vi "Lift.vi"(0 "LiftLocation":T1(ring)) -> ()   [LabVIEW 2018]
uses:
  <vilib>/Rock Robotics/SystemInterfaces/DIO/FPGA_DIOChannel.ctl
  <vilib>/Rock Robotics/WPI/ThirdParty/Phoenix-LabVIEW/Motor Controller/Controls/CTRE_Phoenix_MotorControl_ControlMode.ctl
  Lift Global.vi
  Times/Times Global.vi
  <vilib>/addons/control/pid/pid.llb/PID (DBL).vi
  <vilib>/Rock Robotics/WPI/ThirdParty/Phoenix-LabVIEW/Motor Controller/Get/CTRE_Phoenix_MotorController_GetSelectedSensorData.vi
  Cargo Intake/Cargo Intake Global.vi
  <vilib>/addons/control/pid/NI_PID_pid.lvlib
panel:
  in  "Output Scalar":dbl=0.6 format="%#_13g"
  in  "t":dbl=0.6 format="%#_13g"
  in  "output range":cluster{"output high":dbl, "output low":dbl}={"output high"=1.0, "output low"=-1.0}
  in  "LiftMode":T2(ring)=enum."Basic Control"
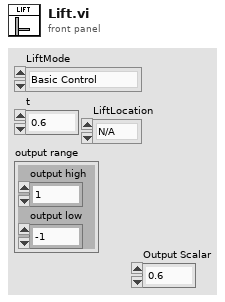
[diagram p1: front panel]
types:
  T1 = enum16{"N/A", "Hatch Panel Zone 1", "Hatch Panel Zone 2", "Hatch Panel Zone 3", "Cargo Zone 1", "Cargo Zone 2", "Cargo Zone 3"}
  T2 = enum16{"Ultra Manual Control", "Manual Control", "Basic Control", "Automated Control", "Autonomous Control"}
  T3 = typedef "FPGA_DIOChannel.ctl" = enum8{"DIO 0", "DIO 1", "DIO 2", "DIO 3", "DIO 4", "DIO 5", "DIO 6", "DIO 7", "DIO 8", "DIO 9", "DIO MXP 0", "DIO MXP 1", "DIO MXP 2", "DIO MXP 3", "DIO MXP 4", "DIO MXP 5", "DIO MXP 6", "DIO MXP 7", "DIO MXP 8", "DIO MXP 9", "DIO MXP 10", "DIO MXP 11", "DIO MXP 12", "DIO MXP 13", "DIO MXP 14", "DIO MXP 15", "SPI Port CS1", "SPI Port CS2", "SPI Port CS3", "SPI Port MISO", "SPI Port MOSI", "Invalid"}
  T4 = typedef "WPI_DigitalInputDevRef.ctl" = cluster{"DevStatus":errorcluster, "DIO Channel":T3}
  T5 = typedef "WPI_MotorControlDeviceRef.ctl" = cluster{"DeviceStatus":errorcluster, "Type":T6, "PWM":cluster{"PWM Channel":T7, "DeadBand":T8}, "CAN":cluster{"Device Number":u8, "SetOutput VI Ref":variant, "GetOutput VI Ref":variant, "Enable VI Ref":variant, "Disable VI Ref":variant, "Data":variant}, "Invert":bool, "DIO PWM":cluster{"PWM \"Enable\" Channel":T7, "DIOChannel":T3, "PWM Rate":dbl}}
  T6 = typedef "WPI_MotorControlType.ctl" = enum16{"PWM", "CAN", "DIO PWM"}
  T7 = typedef "FPGA_DIOPWMChannel.ctl" = enum8{"PWM 0", "PWM 1", "PWM 2", "PWM 3", "PWM 4", "PWM 5", "PWM 6", "PWM 7", "PWM 8", "PWM 9", "PWM MXP 0", "PWM MXP 1", "PWM MXP 2", "PWM MXP 3", "PWM MXP 4", "PWM MXP 5", "PWM MXP 6", "PWM MXP 7", "PWM MXP 8", "PWM MXP 9", "Invalid"}
  T8 = typedef "WPI_PWMDeadband.ctl" = cluster{"Name":string, "maxPositivePwm":i32, "minPositivePwm":i32, "centerPwm":i32, "maxNegativePwm":i32, "minNegativePwm":i32, "angularRange":u16}
  T9 = typedef "CTRE_Phoenix_MotorControl_ControlMode.ctl" = u16
  T10 = typedef "Control 3.ctl" = dbl
  T11 = cluster{"proportional gain (Kc)":dbl, "integral time(Ti, min)":dbl, "derivative time(Td, min) 2":dbl}
  T12 = enum16{"Hatch Panel Zone 1", "Hatch Panel Zone 2", "Hatch Panel Zone 3", "Cargo Zone 1", "Cargo Zone 2", "Cargo Zone 3", "Cargo Ship Zone"}
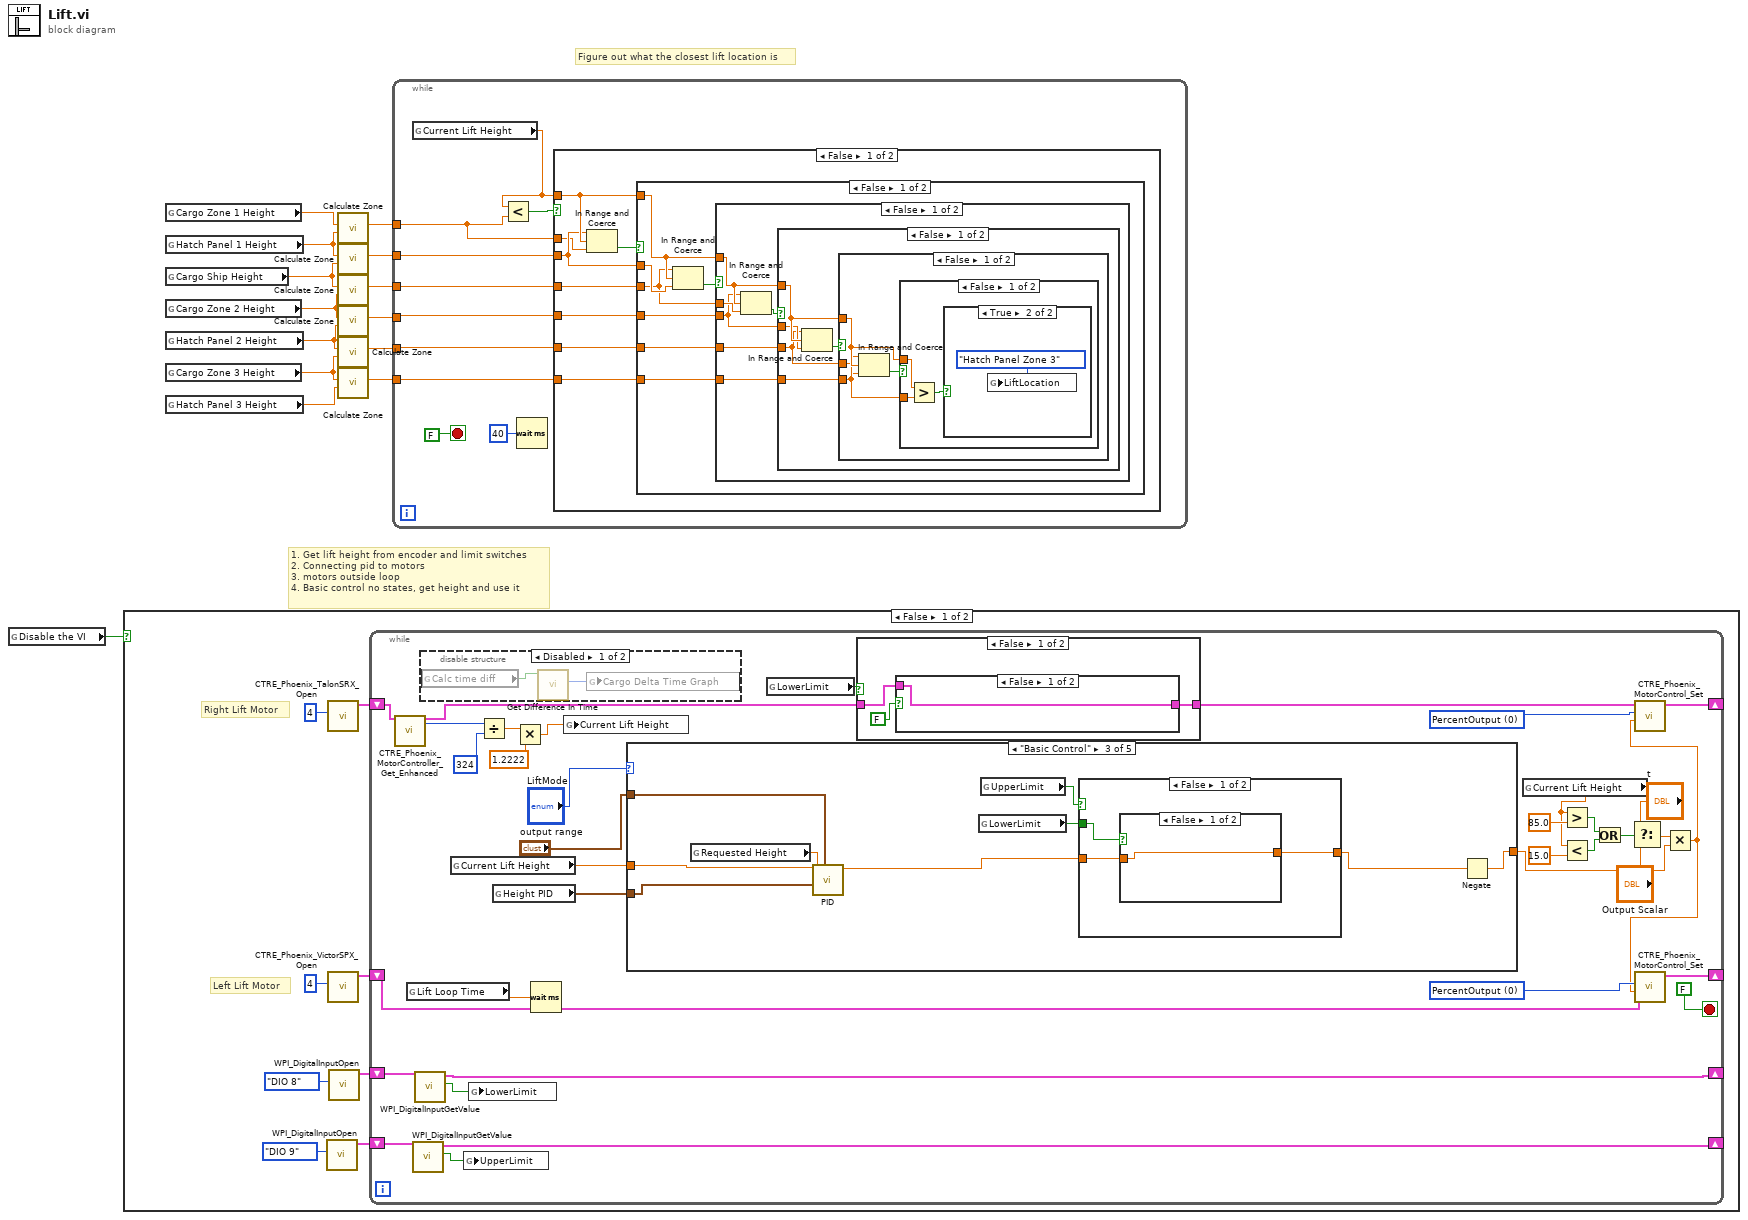
[diagram p0: block diagram]
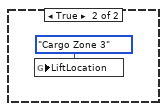
[diagram p3: hidden frame]
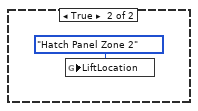
[diagram p4: hidden frame]
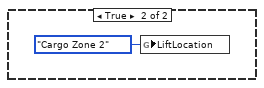
[diagram p5: hidden frame]
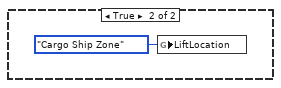
[diagram p6: hidden frame]
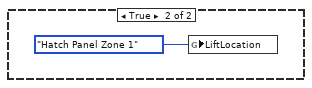
[diagram p7: hidden frame]
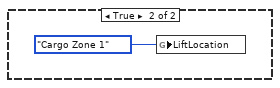
[diagram p8: hidden frame]
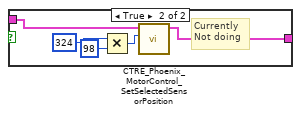
[diagram p9: hidden frame]
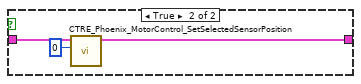
[diagram p10: hidden frame]
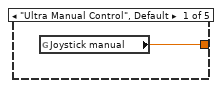
[diagram p12: hidden frame]
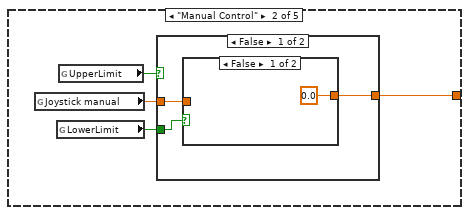
[diagram p13: hidden frame]
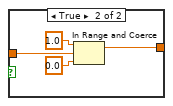
[diagram p14: hidden frame]
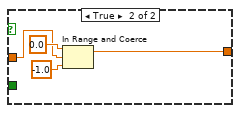
[diagram p15: hidden frame]
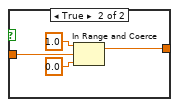
[diagram p16: hidden frame]
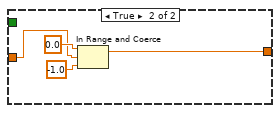
[diagram p17: hidden frame]
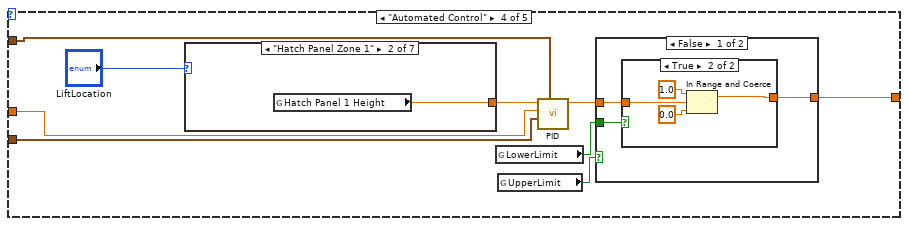
[diagram p18: hidden frame]
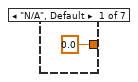
[diagram p19: hidden frame]
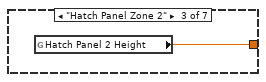
[diagram p20: hidden frame]
diagram:
  # "Figure out what the closest lift location is"
  # "1. Get lift height from encoder and limit switches\n2. Connecting pid to motors\n3. motors outside loop\n4. Basic control no states, get height and use it"
  n1 = global read "Lift Global.vi" "Disable the VI"() -> (w14:bool)
  n2 = case shown="False" w14 {
    frame False {
      # "Left Lift Motor"
      # "Right Lift Motor"
      n3 = call <vilib>:"WPI_DigitalInputOpen.vi"("DIO Channel"=FPGA_DIOChannel."DIO 9") -> ("DigitalInputDevRef"=w15:T4)  [unwired: 9 in, 1 out]
      n4 = call <vilib>:"CTRE_Phoenix_TalonSRX_Open.vi"("Device Number"=u8 4) -> ("CAN Talon SRX Ref"=w22:T5)  [unwired: 9 in, 1 out]
      n5 = call <vilib>:"CTRE_Phoenix_VictorSPX_Open.vi"("Device Number"=u8 4) -> ("CAN Talon SRX Ref"=w20:T5)  [unwired: 9 in, 1 out]
      n6 = call <vilib>:"WPI_DigitalInputOpen.vi"("DIO Channel"=FPGA_DIOChannel."DIO 8") -> ("DigitalInputDevRef"=w17:T4)  [unwired: 9 in, 1 out]
      n7 = while {
        shift-right: [w55] -> _
        shift-left: w22 -> [w48]
        shift-right: [w53] -> _
        shift-left: w20 -> [w52]
        shift-right: [w42] -> _
        shift-left: w17 -> [w43]
        shift-right: [w37] -> _
        shift-left: w15 -> [w38]
        stop <- FALSE stop-if-true
        w54 = T9 0 items=["PercentOutput"=0, "Position"=1, "Velocity"=2, "Current"=3, "Follower"=5, "MotionProfile"=6, "MotionMagic"=7, "MotionProfileArc"=10, "Disabled"=15] ("Control Mode")
        w56 = T9 0 items=["PercentOutput"=0, "Position"=1, "Velocity"=2, "Current"=3, "Follower"=5, "MotionProfile"=6, "MotionMagic"=7, "MotionProfileArc"=10, "Disabled"=15] ("Control Mode")
        n8 = call-poly <vilib>:"CTRE_Phoenix_MotorController_Get_Enhanced.vi"("PhoenixMotorControlDevRef"=w48) -> ("PhoenixMotorControlDevRef"=w47:T5, "Position (Raw Sensor Units)"=w45:i32)  [unwired: 11 in, 2 out]
        n9 = global read "Times Global.vi" "Lift Loop Time"() -> (w59:T10)
        n10 = call <vilib>:"WPI_DigitalInputGetValue.vi"("DigitalInputDevRef"=w38) -> ("Value"=w40:bool, "DigitalInputDevRef"=w37:T4)  [unwired: 8 in, 1 out]
        n11 = call <vilib>:"WPI_DigitalInputGetValue.vi"("DigitalInputDevRef"=w43) -> ("Value"=w41:bool, "DigitalInputDevRef"=w42:T4)  [unwired: 8 in, 1 out]
        n12 = disable-structure shown="Disabled" {
          frame Disabled {
            n13 = global read "Cargo Intake Global.vi" "Calc time diff"() -> (w73:bool)
            n14 = call "Get Difference In Time.vi"("Calculate Time Difference"=w73) -> ("Delta Time over Time"=w72:u32)  [unwired: 9 in, 1 out]
            n15 = global write "Times Global.vi" "Cargo Delta Time Graph"(w72) -> ()
          }
          frame Enabled {
          }
        }
        n16 = global read "Lift Global.vi" "Current Lift Height"() -> (w49:dbl)
        n17 = global write "Lift Global.vi" "UpperLimit"(w40) -> ()
        n18 = global write "Lift Global.vi" "LowerLimit"(w41) -> ()
        n19 = Divide(x=w45, y=324) -> (x/y=w25:dbl)
        n20 = global read "Lift Global.vi" "Height PID"() -> (w50:T11)
        n21 = Multiply(x=w25, y=1.2222) -> (x*y=w24:dbl)
        n22 = Wait (ms)(milliseconds to wait=w59) -> ()  [unwired: 1 out]
        n23 = global write "Lift Global.vi" "Current Lift Height"(w24) -> ()
        n24 = case shown="\"Basic Control\"" "LiftMode" {
          tunnel: [w74 w75 w95 w117 0.0 ("Cargo Zone 3 Height")] -> w29
          tunnel: w49 -> [_ _ w99 w115 _]
          tunnel: w50 -> [_ _ w98 w114 _]
          tunnel: "output range" -> [_ _ w97 w116 _]
          frame "Ultra Manual Control", Default {
            n25 = global read "Lift Global.vi" "Joystick manual"() -> (w74:dbl)
          }
          frame "Manual Control" {
            n26 = global read "Lift Global.vi" "Joystick manual"() -> (w76:dbl)
            n27 = global read "Lift Global.vi" "LowerLimit"() -> (w78:bool)
            n28 = global read "Lift Global.vi" "UpperLimit"() -> (w77:bool)
            n29 = case shown="False" w77 {
              tunnel: w78 -> [w81 _]
              tunnel: [w80 w88] -> w75
              tunnel: w76 -> [w79 w87]
              frame False {
                n30 = case shown="False" w81 {
                  tunnel: [0.0 w86] -> w80
                  tunnel: w79 -> [_ w83]
                  frame False {
                  }
                  frame True {
                    n31 = In Range and Coerce(upper limit=1.0, x=w83, lower limit=0.0) -> (coerced(x)=w86:dbl)  [unwired: 1 out]
                  }
                }
              }
              frame True {
                n32 = In Range and Coerce(upper limit=0.0, x=w87, lower limit=-1.0) -> (coerced(x)=w88:dbl)  [unwired: 1 out]
              }
            }
          }
          frame "Basic Control" {
            n33 = global read "Lift Global.vi" "Requested Height"() -> (w96:dbl)
            n34 = call-poly <vilib>:"PID.vi"("output range"=w97, "PID gains"=w98, "process variable"=w99, "setpoint"=w96) -> ("output"=w92:dbl)  [unwired: 6 in, 1 out]
            n35 = global read "Lift Global.vi" "LowerLimit"() -> (w94:bool)
            n36 = global read "Lift Global.vi" "UpperLimit"() -> (w93:bool)
            n37 = case shown="False" w93 {
              tunnel: w94 -> [w102 _]
              tunnel: [w101 w109] -> w91
              tunnel: w92 -> [w100 w108]
              frame False {
                n38 = case shown="False" w102 {
                  tunnel: [w103 w107] -> w101
                  tunnel: w100 -> [w103 w104]
                  frame False {
                  }
                  frame True {
                    n39 = In Range and Coerce(upper limit=1.0, x=w104, lower limit=0.0) -> (coerced(x)=w107:dbl)  [unwired: 1 out]
                  }
                }
              }
              frame True {
                n40 = In Range and Coerce(upper limit=0.0, x=w108, lower limit=-1.0) -> (coerced(x)=w109:dbl)  [unwired: 1 out]
              }
            }
            n41 = Negate(x=w91) -> (-x=w95:dbl)
          }
          frame "Automated Control" {
            n42 = case shown="\"Hatch Panel Zone 1\"" "LiftLocation" {
              tunnel: [0.0 ("Cargo Zone 3 Height") w122 w123 w124 w125 w126 w127] -> w112
              frame "N/A", Default {
              }
              frame "Hatch Panel Zone 1" {
                n43 = global read "Lift Global.vi" "Hatch Panel 1 Height"() -> (w122:dbl)
              }
              frame "Hatch Panel Zone 2" {
                n44 = global read "Lift Global.vi" "Hatch Panel 2 Height"() -> (w123:dbl)
              }
              frame "Hatch Panel Zone 3" {
                n45 = global read "Lift Global.vi" "Hatch Panel 3 Height"() -> (w124:dbl)
              }
              frame "Cargo Zone 1" {
                n46 = global read "Lift Global.vi" "Cargo Zone 1 Height"() -> (w125:dbl)
              }
              frame "Cargo Zone 2" {
                n47 = global read "Lift Global.vi" "Cargo Zone 2 Height"() -> (w126:dbl)
              }
              frame "Cargo Zone 3" {
                n48 = global read "Lift Global.vi" "Cargo Zone 3 Height"() -> (w127:dbl)
              }
            }
            n49 = global read "Lift Global.vi" "LowerLimit"() -> (w120:bool)
            n50 = global read "Lift Global.vi" "UpperLimit"() -> (w119:bool)
            n51 = call-poly <vilib>:"PID.vi"("output range"=w116, "PID gains"=w114, "process variable"=w115, "setpoint"=w112) -> ("output"=w118:dbl)  [unwired: 6 in, 1 out]
            n52 = case shown="False" w119 {
              tunnel: w120 -> [w130 _]
              tunnel: [w129 w137] -> w117
              tunnel: w118 -> [w128 w136]
              frame False {
                n53 = case shown="True" w130 {
                  tunnel: [0.0 w135] -> w129
                  tunnel: w128 -> [_ w132]
                  frame False {
                  }
                  frame True {
                    n54 = In Range and Coerce(upper limit=1.0, x=w132, lower limit=0.0) -> (coerced(x)=w135:dbl)  [unwired: 1 out]
                  }
                }
              }
              frame True {
                n55 = In Range and Coerce(upper limit=0.0, x=w136, lower limit=-1.0) -> (coerced(x)=w137:dbl)  [unwired: 1 out]
              }
            }
          }
          frame "Autonomous Control" {
          }
        }
        n56 = global read "Lift Global.vi" "LowerLimit"() -> (w39:bool)
        n57 = case shown="False" w39 {
          tunnel: w47 -> [w62 w71]
          tunnel: [w61 w70] -> w46
          frame False {
            n58 = case shown="False" FALSE {
              tunnel: w62 -> [w63 w68]
              tunnel: [w63 w67] -> w61
              frame False {
              }
              frame True {
                # "Currently\nNot doing"
                n59 = Multiply(x=324 ("y"), y=98 ("New Sensor Position")) -> (x*y=w64:i32)
                n60 = call <vilib>:"CTRE_Phoenix_MotorControl_SetSelectedSensorPosition.vi"("New Sensor Position"=w64, "PhoenixMotorControlDevRef"=w68) -> ("PhoenixMotorControlDevRef"=w67:T5)  [unwired: 8 in, 1 out]
              }
            }
          }
          frame True {
            n61 = call <vilib>:"CTRE_Phoenix_MotorControl_SetSelectedSensorPosition.vi"("New Sensor Position"=0, "PhoenixMotorControlDevRef"=w71) -> ("PhoenixMotorControlDevRef"=w70:T5)  [unwired: 8 in, 1 out]
          }
        }
        n62 = global read "Lift Global.vi" "Current Lift Height"() -> (w34:dbl)
        n63 = Greater?(x=w34, y=85.0) -> (0:w32:bool)
        n64 = Less?(x=w34, y=15.0) -> (x < y?=w33:bool)
        n65 = Or(x=w32, y=w33) -> (x .or. y?=w31:bool)
        n66 = Select(t="t", s=w31, f="Output Scalar") -> (s? t:f=w30:dbl)
        n67 = Multiply(x=w30, y=w29) -> (x*y=w26:dbl)
        n68 = call <vilib>:"CTRE_Phoenix_MotorControl_Set.vi"("Output"=w26, "Control Mode"=w56, "PhoenixMotorControlDevRef"=w46) -> ("PhoenixMotorControlDevRef"=w55:T5)  [unwired: 7 in, 1 out]
        n69 = call <vilib>:"CTRE_Phoenix_MotorControl_Set.vi"("Output"=w26, "Control Mode"=w54, "PhoenixMotorControlDevRef"=w52) -> ("PhoenixMotorControlDevRef"=w53:T5)  [unwired: 7 in, 1 out]
      }
    }
    frame True {
    }
  }
  n70 = global read "Lift Global.vi" "Cargo Zone 1 Height"() -> (w7:dbl)
  n71 = global read "Lift Global.vi" "Hatch Panel 1 Height"() -> (w13:dbl)
  n72 = global read "Lift Global.vi" "Cargo Ship Height"() -> (w12:dbl)
  n73 = global read "Lift Global.vi" "Cargo Zone 2 Height"() -> (w11:dbl)
  n74 = global read "Lift Global.vi" "Hatch Panel 2 Height"() -> (w10:dbl)
  n75 = global read "Lift Global.vi" "Cargo Zone 3 Height"() -> (w9:dbl)
  n76 = global read "Lift Global.vi" "Hatch Panel 3 Height"() -> (w8:dbl)
  n77 = call "Calculate Zone.vi"("Top Height"=w13, "Bottom Height"=w7) -> ("Midpoint"=w6:dbl)  [unwired: 9 in]
  n78 = call "Calculate Zone.vi"("Top Height"=w12, "Bottom Height"=w13) -> ("Midpoint"=w5:dbl)  [unwired: 9 in]
  n79 = call "Calculate Zone.vi"("Top Height"=w11, "Bottom Height"=w12) -> ("Midpoint"=w4:dbl)  [unwired: 9 in]
  n80 = call "Calculate Zone.vi"("Top Height"=w10, "Bottom Height"=w11) -> ("Midpoint"=w3:dbl)  [unwired: 9 in]
  n81 = call "Calculate Zone.vi"("Top Height"=w9, "Bottom Height"=w10) -> ("Midpoint"=w2:dbl)  [unwired: 9 in]
  n82 = call "Calculate Zone.vi"("Top Height"=w8, "Bottom Height"=w9) -> ("Midpoint"=w1:dbl)  [unwired: 9 in]
  n83 = while {
    tunnel: w6 -> [w146]
    tunnel: w5 -> [w145]
    tunnel: w4 -> [w144]
    tunnel: w3 -> [w143]
    tunnel: w2 -> [w142]
    tunnel: w1 -> [w141]
    stop <- FALSE stop-if-true
    n84 = global read "Lift Global.vi" "Current Lift Height"() -> (w147:dbl)
    n85 = Less?(x=w147, y=w146) -> (x < y?=w148:bool)
    n86 = Wait (ms)(milliseconds to wait=u32 40) -> ()  [unwired: 1 out]
    n87 = case shown="False" w148 {
      tunnel: w147 -> [w154 _]
      tunnel: w146 -> [w152 _]
      tunnel: w145 -> [w153 _]
      tunnel: w144 -> [w158 _]
      tunnel: w143 -> [w157 _]
      tunnel: w142 -> [w156 _]
      tunnel: w141 -> [w155 _]
      frame False {
        n88 = In Range and Coerce(upper limit=w153, x=w154, lower limit=w152) -> (In Range?=w151:bool)  [unwired: 1 out]
        n89 = case shown="False" w151 {
          tunnel: w154 -> [w161 _]
          tunnel: w153 -> [w160 _]
          tunnel: w158 -> [w159 _]
          tunnel: w157 -> [w165 _]
          tunnel: w156 -> [w164 _]
          tunnel: w155 -> [w163 _]
          frame False {
            n90 = In Range and Coerce(upper limit=w159, x=w161, lower limit=w160) -> (In Range?=w162:bool)  [unwired: 1 out]
            n91 = case shown="False" w162 {
              tunnel: w161 -> [w168 _]
              tunnel: w165 -> [w166 _]
              tunnel: w164 -> [w171 _]
              tunnel: w163 -> [w170 _]
              tunnel: w159 -> [w167 _]
              frame False {
                n92 = In Range and Coerce(upper limit=w166, x=w168, lower limit=w167) -> (In Range?=w169:bool)  [unwired: 1 out]
                n93 = case shown="False" w169 {
                  tunnel: w168 -> [w174 _]
                  tunnel: w171 -> [w172 _]
                  tunnel: w170 -> [w176 _]
                  tunnel: w166 -> [w173 _]
                  frame False {
                    n94 = In Range and Coerce(upper limit=w172, x=w174, lower limit=w173) -> (In Range?=w175:bool)  [unwired: 1 out]
                    n95 = case shown="False" w175 {
                      tunnel: w174 -> [w179 _]
                      tunnel: w176 -> [w178 _]
                      tunnel: w172 -> [w177 _]
                      frame False {
                        n96 = In Range and Coerce(upper limit=w178, x=w179, lower limit=w177) -> (In Range?=w180:bool)  [unwired: 1 out]
                        n97 = case shown="False" w180 {
                          tunnel: w179 -> [w183 _]
                          tunnel: w178 -> [w182 _]
                          frame False {
                            n98 = Greater?(x=w183, y=w182) -> (0:w181:bool)
                            n99 = case shown="True" w181 {
                              frame False {
                              }
                              frame True {
                                n100 = global write "Lift Global.vi" "LiftLocation"(T12."Hatch Panel Zone 3" ("LiftLocation")) -> ()
                              }
                            }
                          }
                          frame True {
                            n101 = global write "Lift Global.vi" "LiftLocation"(T12."Cargo Zone 3" ("LiftLocation")) -> ()
                          }
                        }
                      }
                      frame True {
                        n102 = global write "Lift Global.vi" "LiftLocation"(T12."Hatch Panel Zone 2" ("LiftLocation")) -> ()
                      }
                    }
                  }
                  frame True {
                    n103 = global write "Lift Global.vi" "LiftLocation"(T12."Cargo Zone 2" ("LiftLocation")) -> ()
                  }
                }
              }
              frame True {
                n104 = global write "Lift Global.vi" "LiftLocation"(T12."Cargo Ship Zone" ("LiftLocation")) -> ()
              }
            }
          }
          frame True {
            n105 = global write "Lift Global.vi" "LiftLocation"(T12."Hatch Panel Zone 1" ("LiftLocation")) -> ()
          }
        }
      }
      frame True {
        n106 = global write "Lift Global.vi" "LiftLocation"(T12."Cargo Zone 1" ("LiftLocation")) -> ()
      }
    }
  }
